vi "Move Group Position.vi"(7 "Up (T) / Down (F)":bool, 8 "error in (no error)":errorcluster, 11 "Cfg Grandmaster in":refnum<class "Cfg Grandmaster.lvclass">) -> (0 "error out":errorcluster, 3 "Cfg Grandmaster out":refnum<class "Cfg Grandmaster.lvclass">)   [LabVIEW 2012, in "Configuration Grandmaster.lvlib" / "Cfg Grandmaster.lvclass"]
uses:
  Cfg Grandmaster.lvclass
  Cfg Grandmaster.lvclass/Cfg Grandmaster.ctl
  Class Chassis Cfg/ChassisCfg.lvclass
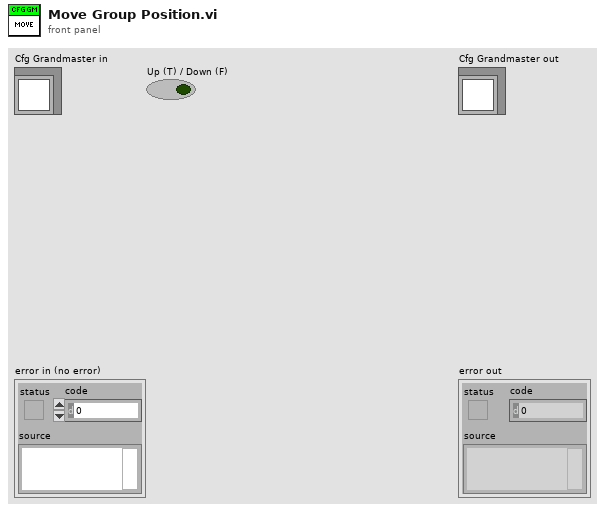
[diagram p1: front panel]
types:
  T1 = typedef "ge_Cfg wChassis.ctl" = cluster{"Chassis BOM":refnum<class "Chassis BOM.lvclass">, "Chassis Cfg":refnum<class "ChassisCfg.lvclass">, "Chassis Tasks":refnum<class "Chassis Tasks.lvclass">, "HW Error":bool, "Unsvd Chgs?":bool}
  T2 = typedef "Selected Group.ctl" = cluster{"ChanGroup":i32, "Rate Class":T3}
  T3 = typedef "TE_Designator.ctl" = enum16{"High Speed", "Low Speed"}
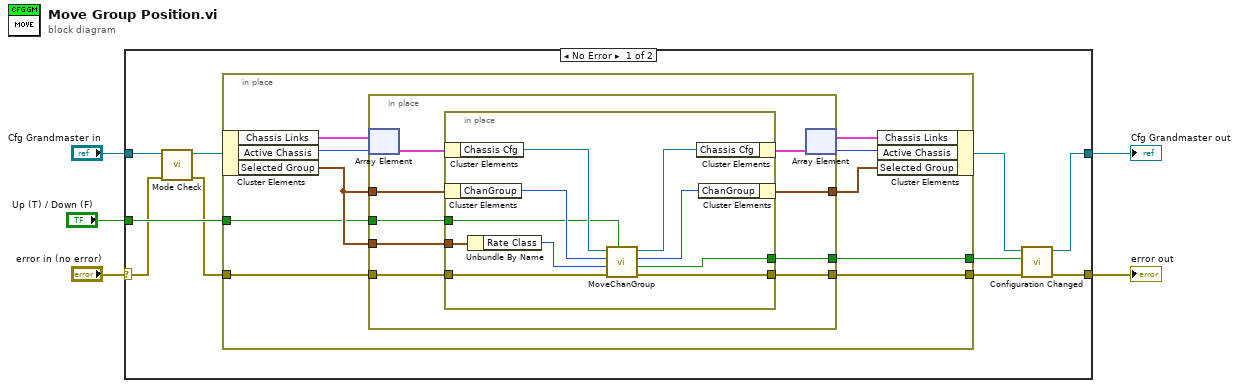
[diagram p0: block diagram]
diagram:
  n1 = case shown="No Error" "error in (no error)" {
    selector: "error in (no error)" -> [w12 w46]
    tunnel: [w9 w46] -> w4
    tunnel: [w8 w45] -> w2
    tunnel: "Cfg Grandmaster in" -> [w14 w45]
    tunnel: "Up (T) / Down (F)" -> [w15 _]
    frame No Error {
      n2 = call "Mode Check.vi"("error in (no error)"=w12, "Cfg Grandmaster in"=w14) -> ("error out"=w11:errorcluster, "Cfg Grandmaster out"=w13:refnum<class "Cfg Grandmaster.lvclass">)  [unwired: 8 in]
      n3 = in-place {
        in-place-border: w11 -> [w21]
        in-place-border: [w20] -> w10
        in-place-border: [w19] -> w6
        in-place-border: w15 -> [w16]
        n4 = in-place-cluster #1(w13) -> ("Chassis Links"=w25:T1[], "Active Chassis"=w24:i32, "Selected Group"=w18:T2)
        n5 = in-place {
          in-place-border: w18 -> [w34]
          in-place-border: [w31] -> w19
          in-place-border: w21 -> [w33]
          in-place-border: [w32] -> w20
          in-place-border: w18 -> [w28]
          in-place-border: [w27] -> w17
          in-place-border: w16 -> [w26]
          n6 = in-place-array #2(w25, w24) -> (w30:T1)
          n7 = in-place {
            in-place-border: w34 -> [w44]
            in-place-border: w33 -> [w43]
            in-place-border: [w42] -> w32
            in-place-border: [w40] -> w31
            in-place-border: w26 -> [w35]
            n8 = in-place-cluster #3(w30) -> ("Chassis Cfg"=w39:refnum<class "ChassisCfg.lvclass">)
            n9 = in-place-cluster #4(w28) -> ("ChanGroup"=w37:i32)
            n10 = Unbundle By Name(w44) -> ("Rate Class"=w41:T3)
            n11 = call "MoveChanGroup.vi"("Up (T) / Down (F)"=w35, "error in (no error)"=w43, "Rate Class"=w41, "ChanGroup"=w37, "Chassis Cfg"=w39) -> ("error out"=w42:errorcluster, "Disregard"=w40:bool, "ChanGroup Out"=w36:i32, "Chassis Cfg"=w38:refnum<class "ChassisCfg.lvclass">)  [unwired: 3 in]
            n12 = in-place-cluster #3("Chassis Cfg"=w38) -> (w29:T1)
            n13 = in-place-cluster #4("ChanGroup"=w36) -> (w27:T2)
          }
          n14 = in-place-array #2(w29) -> (w23:T1[], w22:i32)
        }
        n15 = in-place-cluster #1("Chassis Links"=w23, "Active Chassis"=w22, "Selected Group"=w17) -> (w7:refnum<class "Cfg Grandmaster.lvclass">)
      }
      n16 = call "Configuration Changed.vi"("error in (no error)"=w10, "Canceled? (F)"=w6, "Cfg Grandmaster in"=w7) -> ("error out"=w9:errorcluster, "Cfg Grandmaster out"=w8:refnum<class "Cfg Grandmaster.lvclass">)  [unwired: 7 in]
    }
    frame Error {
    }
  }
  "error out" <- w4
  "Cfg Grandmaster out" <- w2
